vi "Launch Handler.vi"(6 "UUID":string, 8 "Data Model":refnum<class "Device Data Model.lvclass">, 10 "connection reference":refnum<data-value>, 11 "TCP slave":refnum<class "TCP Slave.lvclass">) -> (0 "error out":errorcluster)   [LabVIEW 2021, in "TCP Slave.lvclass"]
doc: "Asynchronously launches a connection handler."
uses:
  TCP Slave.lvclass
  Data Model/Device Data Model.lvclass
  Connection.ctl
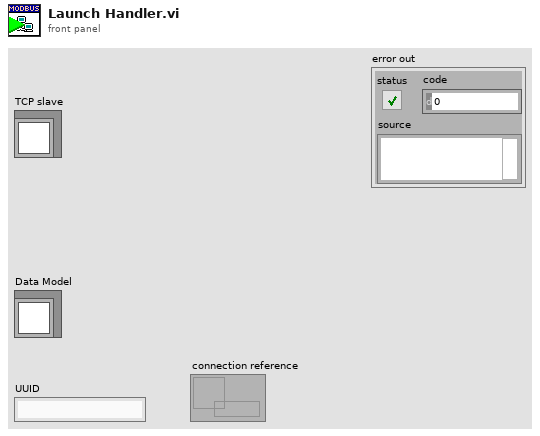
[diagram p1: front panel]
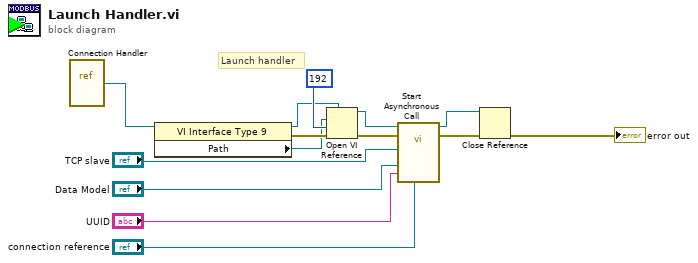
[diagram p0: block diagram]
diagram:
  # "Launch handler"
  n1 = vi-ref "Connection Handler.vi"() -> (w14:refnum<vi>)
  n2 = property class="VI Interface Type 9"(reference=w14) -> (reference out=w1:refnum<vi>, error out=w13:errorcluster, "Path"=w11:path)  [unwired: 1 in]
  n3 = Open VI Reference(type specifier VI Refnum (for type only)=w1, vi path=w11, options=192 ("x .or. y?"), error in (no error)=w13) -> (vi reference=w9:refnum<vi>, error out=w10:errorcluster)  [unwired: 2 in]
  n4 = call-by-ref "Start Asynchronous Call"(reference=w9, error in=w10, "connection reference"="connection reference", "UUID"="UUID", "Data Model"="Data Model", "TCP slave"="TCP slave") -> (reference out=w2:refnum<vi>, error out=w4:errorcluster)  [unwired: 8 in]
  n5 = Close Reference(reference=w2, error in (no error)=w4) -> (error out=→"error out":errorcluster)
